vi "draw_faux_worm.vi"(7 "error in (no error)":errorcluster, 9 "Worms to Draw":T2[](array[typedef]), 10 "Image in":T1) -> (0 "error out":errorcluster, 3 "Image out":T1)   [LabVIEW 2019]
uses:
  <vilib>/vision/Image Controls.llb/IMAQ Image.ctl
  FauxWorm.ctl
  ParametersGlobal.vi
  <vilib>/vision/NI_Vision_Development_Module.lvlib
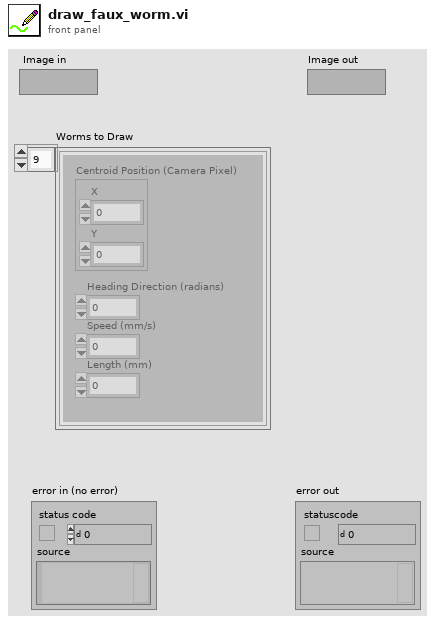
[diagram p1: front panel]
types:
  T1 = typedef "IMAQ Image.ctl" = refnum<image>
  T2 = typedef "FauxWorm.ctl" = cluster{"Centroid Position (Camera Pixel)":cluster{"X":sgl, "Y":sgl}, "Heading Direction (radians)":dbl, "Speed (mm/s)":sgl, "Length (mm)":sgl}
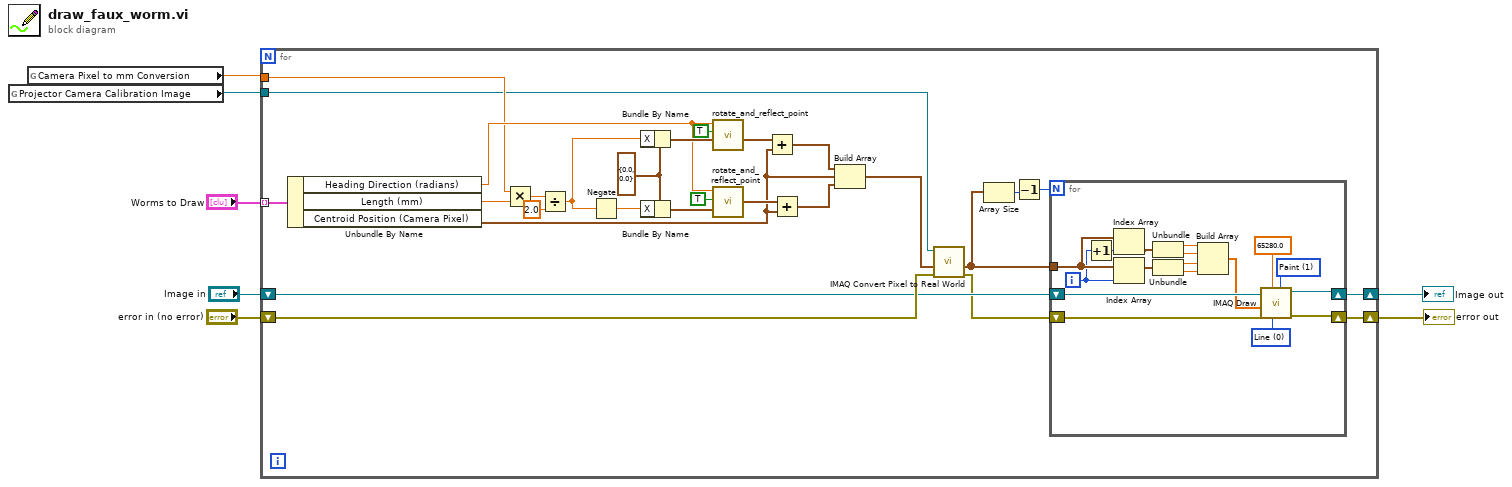
[diagram p0: block diagram]
diagram:
  n1 = global read "ParametersGlobal.vi" "Projector Camera Calibration Image"() -> (w2:T1)
  n2 = global read "ParametersGlobal.vi" "Camera Pixel to mm Conversion"() -> (w1:sgl)
  n3 = for {
    tunnel: "Worms to Draw" -> [w35] mode=indexing
    shift-right: [w11] -> w4
    shift-left: "Image in" -> [w16]
    shift-right: [w10] -> w3
    shift-left: "error in (no error)" -> [w34]
    tunnel: w1 -> [w9]
    tunnel: w2 -> [w8]
    w28 = cluster{"X":sgl, "Y":sgl} {"X"=0.0, "Y"=0.0} ("Centroid Position (Camera Pixel)")
    n4 = Unbundle By Name(w35) -> ("Heading Direction (radians)"=w26:dbl, "Length (mm)"=w33:sgl, "Centroid Position (Camera Pixel)"=w17:cluster{"X":sgl, "Y":sgl})
    n5 = Multiply(x=w9, y=w33) -> (x*y=w32:sgl)
    n6 = Divide(x=w32, y=sgl 2.0) -> (x/y=w29:sgl)
    n7 = Negate(x=w29) -> (-x=w30:sgl)
    n8 = Bundle By Name(cluster=w28, "X"=w29) -> (w27:cluster{"X":sgl, "Y":sgl})
    n9 = Bundle By Name(cluster=w28, "X"=w30) -> (w25:cluster{"X":sgl, "Y":sgl})
    n10 = call "rotate_and_reflect_point.vi"("Point"=w27, "reflect about the x axis?"=TRUE, "rotation angle (radians)"=w26) -> ("transformed point"=w23:cluster{"X":sgl, "Y":sgl})  [unwired: 8 in]
    n11 = call "rotate_and_reflect_point.vi"("Point"=w25, "reflect about the x axis?"=TRUE, "rotation angle (radians)"=w26) -> ("transformed point"=w24:cluster{"X":sgl, "Y":sgl})  [unwired: 8 in]
    n12 = Add(x=w23, y=w17) -> (x+y=w22:cluster{"X":sgl, "Y":sgl})
    n13 = Add(x=w24, y=w17) -> (x+y=w21:cluster{"X":sgl, "Y":sgl})
    n14 = Build Array(w22, w17, w21) -> (w20:cluster{"X":sgl, "Y":sgl}[])
    n15 = call "IMAQ Convert Pixel to Real World"("error in (no error)"=w34, "Array of Pixel Coordinates"=w20, "Calibrated Image"=w8) -> ("error out"=w12:errorcluster, "Array of Real World Coordinates"=w13:cluster{"X":sgl, "Y":sgl}[])  [unwired: 3 in, 4 out]
    n16 = Array Size(array=w13) -> (size(s)=w15:i32)
    n17 = Decrement(x=w15) -> (x-1=w14:i32)
    n18 = for {
      N: w14 -> [_]
      shift-right: [w49] -> w11
      shift-left: w16 -> [w50]
      tunnel: w13 -> [w48]
      shift-right: [w37] -> w10
      shift-left: w12 -> [w38]
      i -> [w46]
      w51 = u16 1 items=["Frame", "Paint", "Invert Frame", "Invert Paint"] ("Draw Mode")
      w52 = u16 0 items=["Line", "Rectangle", "Oval"] ("Shape to draw")
      n19 = Increment(x=w46) -> (x+1=w47:i32)
      n20 = Index Array(array=w48, index=w47) -> (element=w45:cluster{"X":sgl, "Y":sgl})
      n21 = Index Array(array=w48, index=w46) -> (element=w44:cluster{"X":sgl, "Y":sgl})
      n22 = Unbundle(w45) -> ("X"=w43:sgl, "Y"=w42:sgl)
      n23 = Unbundle(w44) -> ("X"=w41:sgl, "Y"=w40:sgl)
      n24 = Build Array(w43, w42, w41, w40) -> (w39:sgl[])
      n25 = call "IMAQ Draw"("Draw Mode"=w51, "Shape to draw"=w52, "Pixel Color"=sgl 65280.0, "error in (no error)"=w38, "Coordinates"=w39, "Image Src"=w50) -> ("error out"=w37:errorcluster, "Image Dst Out"=w49:T1)  [unwired: 4 in]
    }
  }
  "error out" <- w3
  "Image out" <- w4
